vi "AutoAlign_ASI.vi"() -> ()   [LabVIEW 2014]
uses:
  Controls/StageStates.ctl
  Controls/GraphNotifier2D.ctl
panel:
  out "Moving":bool
  in  "Done":bool
  in  "Repeat":bool
  in  "Start":bool
  out "Position":dbl
  in  "Scan Range":dbl=7.0
  out "Intensity Graph":u16[][](graph)
  in  "Quit":bool
  out "Sample":cluster{"X":dbl, "Y":dbl}[](graph)
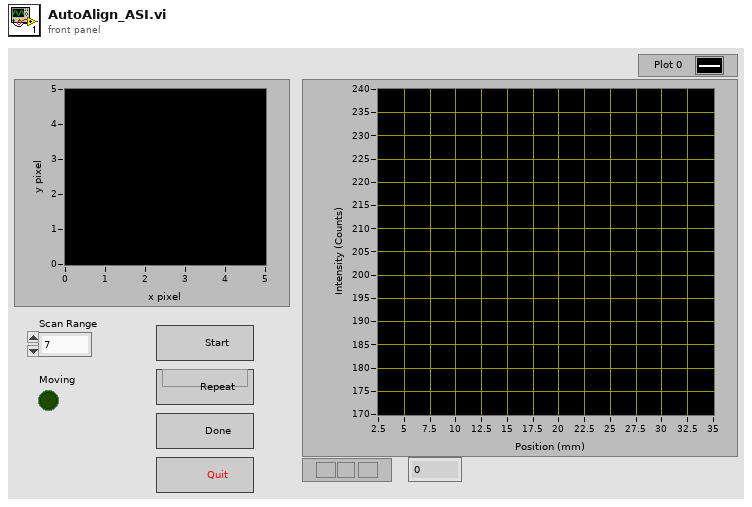
[diagram p1: front panel]
types:
  T1 = typedef "GraphNotifier2D.ctl" = cluster{"Xpos":i32, "Ypos":i32, "subarray":sgl[][], "Intensity":sgl}
  T2 = typedef "LabVIEW Interface for Arduino.lvlib/Arduino Resource.ctl" = cluster{"VISA resource":refnum<visa-resource-name>, "Board Type":T3, "Connection Type":enum8{"USB / Serial"}, "Bytes Per Packet (15)":u8}
  T3 = typedef "LabVIEW Interface for Arduino.lvlib/Board Type.ctl" = enum16{"Uno", "Dimuelanove w/Atmega 328", "Mega 2560"}
  T4 = typedef "StageStates.ctl" = enum16{"POSITION", "MVR", "MOVE", "HALT", "ONTARGET", "ERROR", "EXIT", "HOME", "ZEROPOS", "NANOPOS", "QUIT", "ANALOG"}
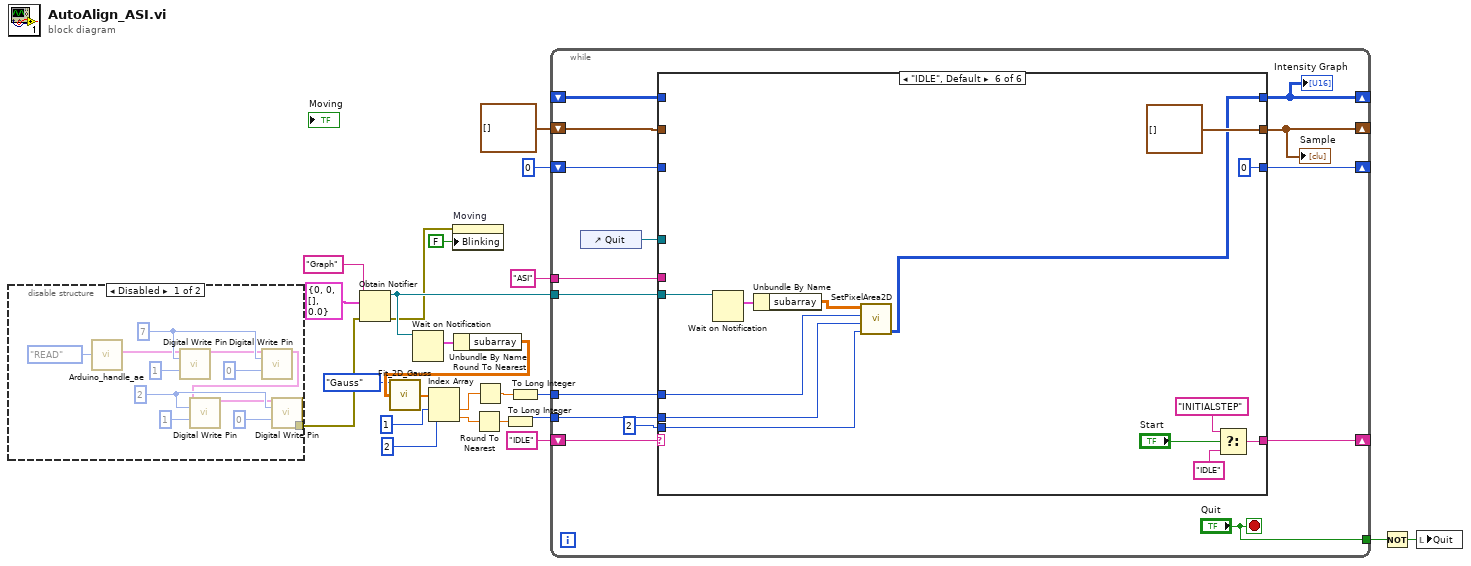
[diagram p0: block diagram]
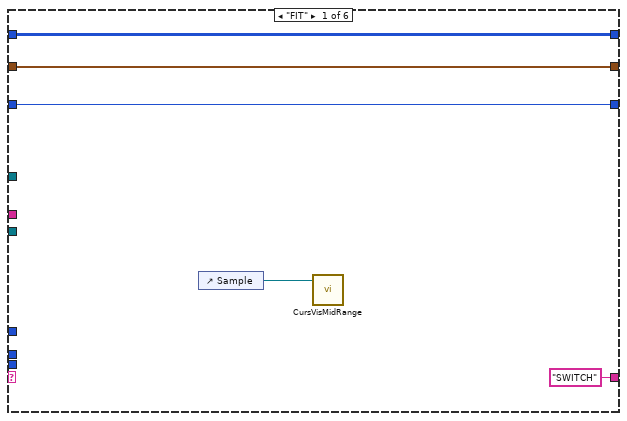
[diagram p3: hidden frame]
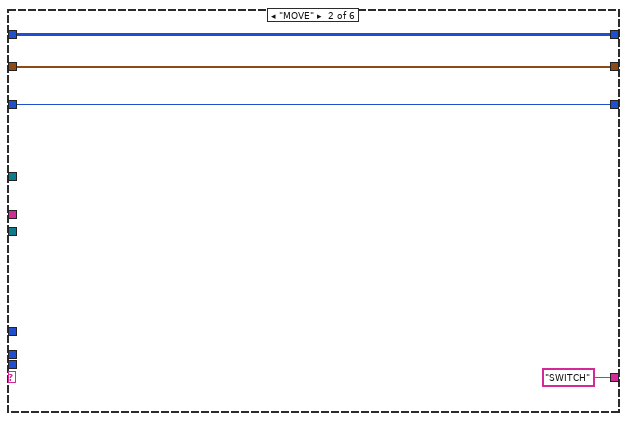
[diagram p4: hidden frame]
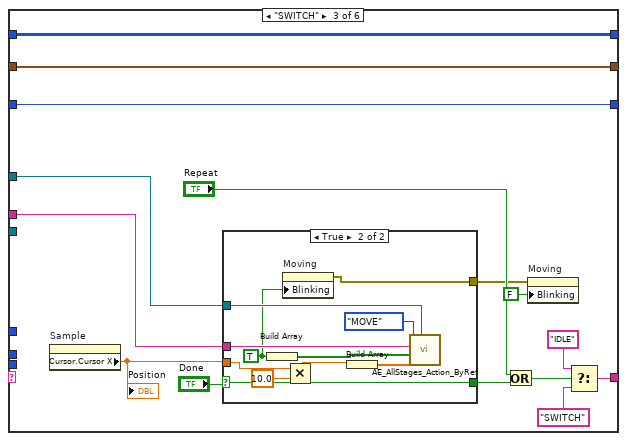
[diagram p5: hidden frame]
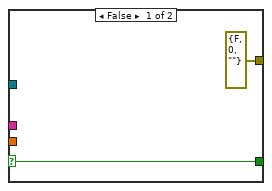
[diagram p6: hidden frame]
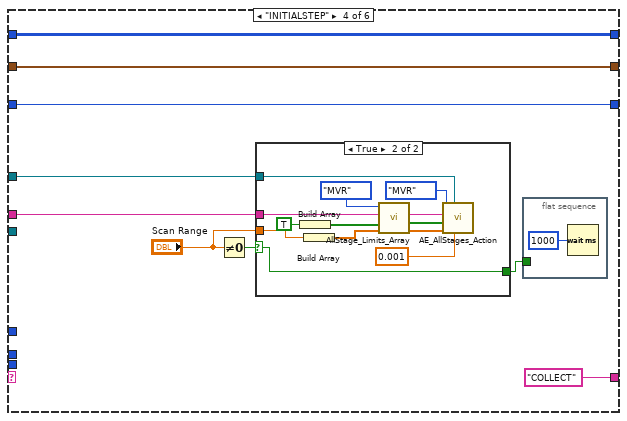
[diagram p7: hidden frame]
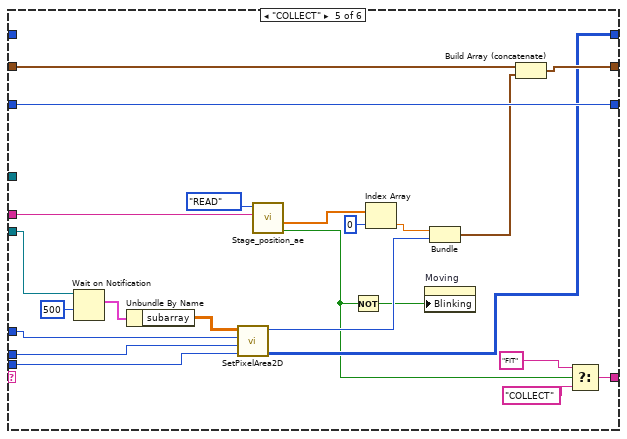
[diagram p9: hidden frame]
diagram:
  n1 = disable-structure shown="Disabled" {
    disable-tunnel: [w25 _] -> w14
    frame Disabled {
      w36 = u8 2 ("Digital I/O Pin (0)")
      w31 = u8 7 ("Digital I/O Pin (0)")
      n2 = call "Arduino_handle_ae.vi"("Enum"=enum16{"WRITE", "READ"}."READ") -> ("Arduino Resource Out"=w30:T2)  [unwired: 10 in]
      n3 = call <vilib>:"Digital Write Pin.vi"("Arduino Resource"=w30, "Digital I/O Pin (0)"=w31, "Value (0)"=u8 1) -> ("Arduino Resource"=w26:T2)  [unwired: 11 in, 1 out]
      n4 = call <vilib>:"Digital Write Pin.vi"("Arduino Resource"=w26, "Digital I/O Pin (0)"=w31, "Value (0)"=u8 0) -> ("Arduino Resource"=w35:T2)  [unwired: 11 in, 1 out]
      n5 = call <vilib>:"Digital Write Pin.vi"("Arduino Resource"=w35, "Digital I/O Pin (0)"=w36, "Value (0)"=u8 1) -> ("Arduino Resource"=w34:T2)  [unwired: 11 in, 1 out]
      n6 = call <vilib>:"Digital Write Pin.vi"("Arduino Resource"=w34, "Digital I/O Pin (0)"=w36, "Value (0)"=u8 0) -> ("error out"=w25:errorcluster)  [unwired: 11 in, 1 out]
    }
    frame Enabled {
    }
  }
  n7 = Obtain Notifier(name (unnamed)="Graph", notification data type=T1 {"Xpos"=0, "Ypos"=0, "subarray"=[], "Intensity"=0.0}, error in (no error)=w14) -> (notifier out=w15:refnum<notifier>, error out=w1:errorcluster)  [unwired: 1 in, 1 out]
  n8 = Wait on Notification(notifier=w15) -> (notification=w16:T1)  [unwired: 3 in, 3 out]
  n9 = property on="Moving" class="Bool (strict)"(error in=w1, "Blinking"=FALSE) -> ()  [unwired: 1 in, 2 out]
  n10 = Unbundle By Name(w16) -> ("subarray"=w13:sgl[][])
  n11 = call "Fit_2D_Gauss.vi"("Enum"=enum16{"Gauss", "Lorentz"}."Gauss", "Image IN"=w13) -> ("Fit Parameters"=w12:dbl[])  [unwired: 12 in, 1 out]
  n12 = Index Array(array=w12, index #1=1 ("index"), index #2=2 ("index")) -> (element #1=w9:dbl, element #2=w8:dbl)
  n13 = Round To Nearest(number=w8) -> (nearest integer value=w6:dbl)
  n14 = Round To Nearest(number=w9) -> (nearest integer value=w7:dbl)
  n15 = To Long Integer(number=w6) -> (32bit integer=w4:i32)
  n16 = To Long Integer(number=w7) -> (32bit integer=w5:i32)
  n17 = while {
    shift-right: [w49] -> _
    shift-left: _ -> [w51]
    shift-right: [w50] -> _
    shift-left: cluster{"x":dbl, "y":dbl}[] [] ("XY chart data") -> [w41]
    shift-right: [w48] -> _
    shift-left: "IDLE" -> [w44]
    shift-right: [w46] -> _
    shift-left: 0 ("NumberOfSteps 2") -> [w47]
    tunnel: w15 -> [w43]
    tunnel: "ASI" ("StageID") -> [w42]
    tunnel: ["Quit"] -> w18
    tunnel: w5 -> [w39]
    tunnel: w4 -> [w38]
    stop <- "Quit" stop-if-true
    n18 = control-ref of="Quit"() -> (w45:refnum<vi>)
    n19 = case shown="\"IDLE\", Default" w44 {
      tunnel: [w56 w60 w73 w97 w116 w137] -> w49
      tunnel: w51 -> [w56 w60 w73 w97 _ _]
      tunnel: w41 -> [w52 w59 w74 w90 w126 _]
      tunnel: [w52 w59 w74 w90 w125 cluster{"x":dbl, "y":dbl}[] [] ("XY chart data")] -> w50
      tunnel: w42 -> [_ _ w70 w91 w128 _]
      tunnel: ["SWITCH" "SWITCH" w67 "COLLECT" w124 w147] -> w48
      tunnel: w47 -> [w55 w58 w75 w96 w135 _]
      tunnel: [w55 w58 w75 w96 w135 0 ("NumberOfSteps 2")] -> w46
      tunnel: w45 -> [_ _ w72 w95 _ _]
      tunnel: w43 -> [_ _ _ _ w129 w142]
      tunnel: w39 -> [_ _ _ _ w119 w139]
      tunnel: w38 -> [_ _ _ _ w118 w138]
      tunnel: 2 ("Area") -> [_ _ _ _ w115 w136]
      frame "FIT" {
        n20 = control-ref of="Sample"() -> (w53:refnum<vi>)
        n21 = call "CursVisMidRange.vi"("XYGraph in"=w53) -> ()  [unwired: 11 in]
      }
      frame "MOVE" {
      }
      frame "SWITCH" {
        n22 = property on="Sample" class="XYGraph (strict)"() -> ("Cursor.Cursor X"=w71:dbl)  [unwired: 2 in, 2 out]
        "Position" <- w71
        n23 = case shown="True" "Done" {
          selector: "Done" -> [w77 w86]
          tunnel: w70 -> [_ w85]
          tunnel: w72 -> [_ w87]
          tunnel: w71 -> [_ w83]
          tunnel: [w77 w86] -> w64
          tunnel: [errorcluster {"status"=FALSE, "code"=0, "source"=""} ("error out") w78] -> w61
          frame False {
          }
          frame True {
            w79 = TRUE
            n24 = Build Array(w79) -> (w84:bool[])
            n25 = property on="Moving" class="Bool (strict)"("Blinking"=w79) -> (error out=w78:errorcluster)  [unwired: 2 in, 1 out]
            n26 = Multiply(x=w83, y=10.0) -> (x*y=w81:dbl)
            n27 = Build Array(w81) -> (w82:dbl[])
            n28 = call "AE_AllStages_Action_ByRef.vi"("Abort"=w87, "Positions"=w82, "Axis"=w84, "Stage ID"=w85, "Action"=StageStates."MOVE") -> ()  [unwired: 3 in, 4 out]
          }
        }
        n29 = Or(x="Repeat", y=w64) -> (x .or. y?=w66:bool)
        n30 = property on="Moving" class="Bool (strict)"(error in=w61, "Blinking"=FALSE) -> ()  [unwired: 1 in, 2 out]
        n31 = Select(t="IDLE", s=w66, f="SWITCH") -> (s? t:f=w67:string)
      }
      frame "INITIALSTEP" {
        n32 = Not Equal To 0?(x="Scan Range") -> (x != 0?=w93:bool)
        n33 = case shown="True" w93 {
          selector: w93 -> [w99 w101]
          tunnel: w91 -> [_ w108]
          tunnel: w95 -> [_ w110]
          tunnel: "Scan Range" -> [_ w109]
          tunnel: [w99 w101] -> w89
          frame False {
          }
          frame True {
            n34 = Build Array(TRUE) -> (w106:bool[])
            n35 = Build Array(w109) -> (w100:dbl[])
            n36 = call "AllStage_Limits_Array.vi"("Step(um)/Position(units)"=w100, "Axis"=w106, "Stage ID"=w108, "MOVE/MVR"=enum16{"MOVE", "MVR"}."MVR") -> ("Positions"=w103:dbl[], "Boolean Array"=w104:bool[], "Stage ID"=w105:string)  [unwired: 5 in]
            n37 = call "AE_AllStages_Action.vi"("Velocity"=0.001, "Abort"=w110, "Positions"=w103, "Axis"=w104, "Stage ID"=w105, "Action"=StageStates."MVR") -> ()  [unwired: 3 in, 3 out]
          }
        }
        n38 = flat-sequence {
          tunnel: w89 -> [_]
          frame #0 {
            n39 = Wait (ms)(milliseconds to wait=u32 1000) -> ()  [unwired: 1 out]
          }
        }
      }
      frame "COLLECT" {
        n40 = Wait on Notification(notifier=w129, timeout in ms (-1)=500) -> (notification=w131:T1)  [unwired: 2 in, 3 out]
        n41 = Unbundle By Name(w131) -> ("subarray"=w120:sgl[][])
        n42 = call "SetPixelArea2D.vi"("Area"=w115, "Y"=w118, "X"=w119, "Array"=w120) -> ("subarray"=w116:u16[][], "AvIntens"=w117:u16)  [unwired: 6 in]
        n43 = call "Stage_position_ae.vi"("StageID"=w128, "Enum"=enum16{"WRITE", "READ"}."READ") -> ("Status Out"=w114:bool, "Position Out"=w133:dbl[])  [unwired: 8 in]
        n44 = Not(x=w114) -> (.not. x?=w113:bool)
        n45 = Index Array(array=w133, index=0) -> (element=w121:dbl)
        n46 = property on="Moving" class="Bool (strict)"("Blinking"=w113) -> ()  [unwired: 2 in, 2 out]
        n47 = Bundle("Numeric"=w121, "AvIntens"=w117) -> (w127:cluster{"Numeric":dbl, "AvIntens":u16})  [unwired: 1 in]
        n48 = Build Array (concatenate)(w126, w127) -> (w125:cluster{"Numeric":dbl, "y":dbl}[])
        n49 = Select(t="FIT", s=w114, f="COLLECT") -> (s? t:f=w124:string)
      }
      frame "IDLE", Default {
        n50 = Wait on Notification(notifier=w142) -> (notification=w143:T1)  [unwired: 3 in, 3 out]
        n51 = Unbundle By Name(w143) -> ("subarray"=w140:sgl[][])
        n52 = call "SetPixelArea2D.vi"("Area"=w136, "Y"=w138, "X"=w139, "Array"=w140) -> ("subarray"=w137:u16[][])  [unwired: 6 in, 1 out]
        n53 = Select(t="INITIALSTEP", s="Start", f="IDLE") -> (s? t:f=w147:string)
      }
    }
    "Sample" <- w50
    "Intensity Graph" <- w49
  }
  n54 = Not(x=w18) -> (.not. x?=w17:bool)
  n55 = local write "Quit"(w17) -> ()
